vi "Configuration Data MHLC.vi"(8 "error in (no error)":errorcluster, 10 "Data in":variant, 11 "Debug Server in":refnum<class "Debug Server.lvclass">) -> (0 "error out":errorcluster, 3 "Debug Server out":refnum<class "Debug Server.lvclass">)   [LabVIEW 2017, in "Debug Server.lvclass"]
doc: "Configuration Data has been returned from the Settings Worker. Send these settings to Application Manager Worker and store the rest in this Worker's shift-register.\nStart the TCP Server listening on the selected Port."
uses:
  Debug Server.lvclass
  C:/Program Files (x86)/National Instruments/LabVIEW 2017/vi.lib/addons/_Workers/Library/Classes/Worker/Worker.lvclass
  Application Manager/rqp_Receive Config Data.ctl
  <vilib>/Utility/miscctls.llb/LVRectTypeDef.ctl
  Debug Server TCP Server and Client/Workers/DS TCP Server/rqp_Start Listening.ctl
  <vilib>/addons/_Workers/Library/Classes/Message Queue/Message Queue.lvclass
  Debug Server.lvclass/Debug Server.ctl
  Application Manager/Application Manager.lvclass
  Settings/Settings.lvclass
  Debug Server TCP Server and Client/Workers/DS TCP Server/DS TCP Server.lvclass
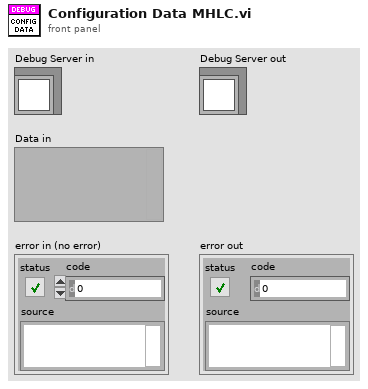
[diagram p1: front panel]
types:
  T1 = typedef "DS TCP Server.lvlib/DS TCP Server.lvclass/rqp_Start Listening.ctl" = cluster{"Server Name":string, "Port":u16, "App Manager Q":refnum<class "Message Queue.lvclass">}
  T2 = typedef "Application Manager.lvclass/rqp_Receive Config Data.ctl" = cluster{"Server Port":u16, "WinBounds":T3, "FP.State":enum32{"Invalid", "Standard", "Closed", "Hidden", "Minimized", "Maximized"}, "Monitor":u16, "Column Widths":u32[]}
  T3 = typedef "LVRectTypeDef.ctl" = cluster{"Left":i16, "Top":i16, "Right":i16, "Bottom":i16}
  T4 = typedef "Settings.lvclass/rsp_Configuration Data.ctl" = cluster{"Config Data":T5}
  T5 = typedef "Settings.lvclass/Config Data.ctl" = cluster{"DS First Launch":bool, "LogBaseFolder":path, "Live Logging":bool, "Server Port":u16, "Max Number ML Rows":i32, "AM.WinBounds":T3, "AM.FP.State":enum32{"Invalid", "Standard", "Closed", "Hidden", "Minimized", "Maximized"}, "AM.Monitor":u16, "AM.Column Widths":u32[], "ML.Visible Columns":bool[], "ML.Splitter Position":i32, "ML.Column Widths":u32[], "ML.WinBounds":T3, "ML.FP.State":enum32{"Invalid", "Standard", "Closed", "Hidden", "Minimized", "Maximized"}, "ML.Monitor":u16}
  T6 = enum32{"Invalid", "Standard", "Closed", "Hidden", "Minimized", "Maximized"}
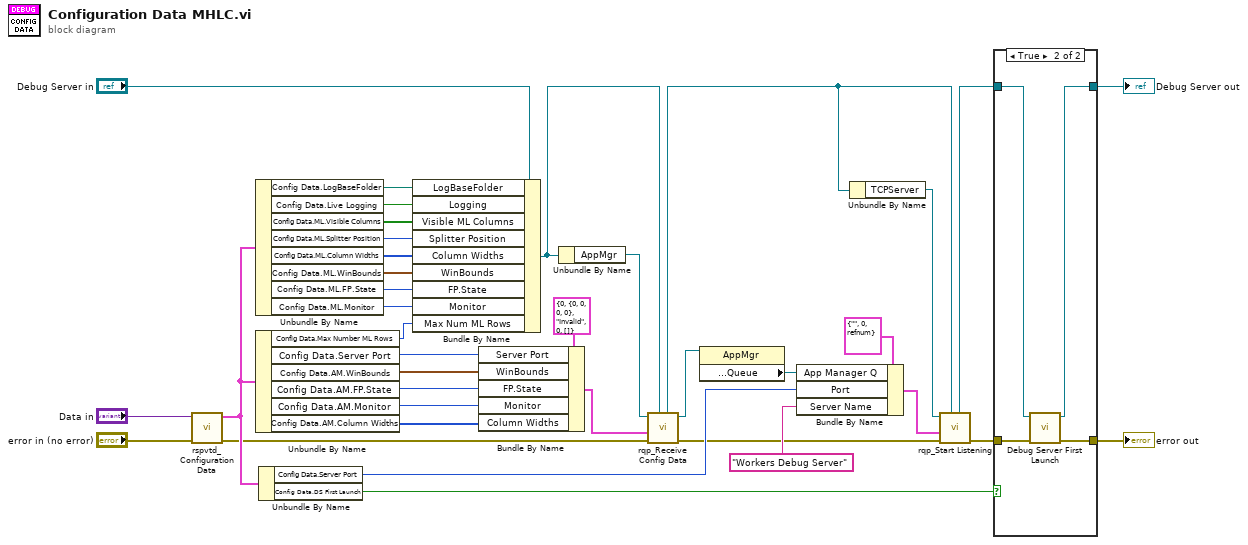
[diagram p0: block diagram]
diagram:
  n1 = call "rspvtd_Configuration Data.vi"("error in"="error in (no error)", "Data in"="Data in") -> ("error out"=w7:errorcluster, "Data out"=w25:T4)  [unwired: 8 in]
  n2 = Unbundle By Name(w25) -> ("Config Data.LogBaseFolder"=w34:path, "Config Data.Live Logging"=w33:bool, "Config Data.ML.Visible Columns"=w26:bool[], "Config Data.ML.Splitter Position"=w27:i32, "Config Data.ML.Column Widths"=w28:u32[], "Config Data.ML.WinBounds"=w29:T3, "Config Data.ML.FP.State"=w30:T6, "Config Data.ML.Monitor"=w31:u16)
  n3 = Unbundle By Name(w25) -> ("Config Data.Max Number ML Rows"=w32:i32, "Config Data.Server Port"=w12:u16, "Config Data.AM.WinBounds"=w13:T3, "Config Data.AM.FP.State"=w14:T6, "Config Data.AM.Monitor"=w15:u16, "Config Data.AM.Column Widths"=w16:u32[])
  n4 = Unbundle By Name(w25) -> ("Config Data.Server Port"=w21:u16, "Config Data.DS First Launch"=w4:bool)
  n5 = Bundle By Name(cluster="Debug Server in", "LogBaseFolder"=w34, "Logging"=w33, "Visible ML Columns"=w26, "Splitter Position"=w27, "Column Widths"=w28, "WinBounds"=w29, "FP.State"=w30, "Monitor"=w31, "Max Num ML Rows"=w32) -> (w24:refnum<class "Debug Server.lvclass">)
  n6 = Bundle By Name(cluster=T2 {"Server Port"=0, "WinBounds"={"Left"=0, "Top"=0, "Right"=0, "Bottom"=0}, "FP.State"=enum."Invalid", "Monitor"=0, "Column Widths"=[]} ("Data"), "Server Port"=w12, "WinBounds"=w13, "FP.State"=w14, "Monitor"=w15, "Column Widths"=w16) -> (w11:T2)
  n7 = Unbundle By Name(w24) -> ("AppMgr"=w3:refnum<class "Application Manager.lvclass">)
  n8 = call "rqp_Receive Config Data.vi"("Caller in"=w24, "error in"=w7, "Data in"=w11, "Application Manager in"=w3) -> ("error out"=w8:errorcluster, "dup Application Manager out"=w1:refnum<class "Application Manager.lvclass">, "dup Caller out"=w18:refnum<class "Debug Server.lvclass">)  [unwired: 5 in]
  n9 = property class="AppMgr"(reference=w1) -> ("Accessors:Read:Public API:Queue"=w2:refnum<class "Message Queue.lvclass">)  [unwired: 1 in, 2 out]
  n10 = Bundle By Name(cluster=T1 {"Server Name"="", "Port"=0, "App Manager Q"=refnum} ("Data in"), "App Manager Q"=w2, "Port"=w21, "Server Name"="Workers Debug Server") -> (w22:T1)
  n11 = Unbundle By Name(w18) -> ("TCPServer"=w19:refnum<class "DS TCP Server.lvclass">)
  n12 = call "rqp_Start Listening.vi"("Caller in"=w18, "error in"=w8, "Data in"=w22, "DS TCP Server in"=w19) -> ("error out"=w17:errorcluster, "dup Caller out"=w36:refnum<class "Debug Server.lvclass">)  [unwired: 5 in, 1 out]
  n13 = case shown="True" w4 {
    tunnel: [w39 w43] -> w37
    tunnel: w36 -> [w39 w42]
    tunnel: [w38 w41] -> w35
    tunnel: w17 -> [w38 w40]
    frame False {
    }
    frame True {
      n14 = call "Debug Server First Launch.vi"("error in (no error)"=w40, "Debug Server in"=w42) -> ("error out"=w41:errorcluster, "Debug Server out"=w43:refnum<class "Debug Server.lvclass">)  [unwired: 8 in]
    }
  }
  "Debug Server out" <- w37
  "error out" <- w35
